vi "publish -- pll result.vi"(7 "publisher action":T4, 11 "pll result IN":T1={"freq (Hz)"=40017.438097734725, "gamma (Hz)"=0.0, "Voltage (V)"=6.817921124952451+0.0i, "overlimit ?"=FALSE, "running lorentzian out"={"A (VHz)"=-1.0311345636926572, "f (Hz)"=-1.0311345636926572, "G (Hz)"=-1.0311345636926572, "phi(rad)"=-1.0311345636926572, "Q"=-1.0311345636926572, "Norm  Ampl"=-1.0311345636926572, "bg (V)"=-1.0311345636926572+0.0i, "4corners"={"z (-pi/2)"=-1.0311345636926572+0.5736824521422934i, "z(inf)"=-0.5200164984937075+1.0975277942502903i, "z (pi/2)"=-1.0311345636926572+0.5736824521422934i, "z center"=-0.5136528600391839+0.580046090596817i, "z(0)"=-0.5200164984937075+1.0975277942502903i, "radius"=-1.0311345636926572}}, "static lorentzian out"={"A (VHz)"=6.817921124952451, "f (Hz)"=-1.0311345636926572, "G (Hz)"=-1.0311345636926572, "phi(rad)"=-1.0311345636926572, "Q"=-1.0311345636926572, "Norm  Ampl"=-1.0311345636926572, "bg (V)"=-1.0311345636926572+0.0i, "4corners"={"z (-pi/2)"=-1.0311345636926572+0.5736824521422934i, "z(inf)"=-0.5200164984937075+1.0975277942502903i, "z (pi/2)"=-1.0311345636926572+0.5736824521422934i, "z center"=-0.5136528600391839+0.580046090596817i, "z(0)"=-0.5200164984937075+1.0975277942502903i, "radius"=-1.0311345636926572}}} {"static lorentzian out"."bg (V)" format="%#9_9f"; "static lorentzian out"."Q" format="%#9_9f"; "static lorentzian out"."phi(rad)" format="%#9_9f"; "static lorentzian out"."G (Hz)" format="%#9_9f"; "static lorentzian out"."f (Hz)" format="%#9_9f"; "running lorentzian out"."bg (V)" format="%#9_9f"; "running lorentzian out"."Q" format="%#9_9f"; "running lorentzian out"."phi(rad)" format="%#9_9f"; "running lorentzian out"."G (Hz)" format="%#9_9f"; "running lorentzian out"."f (Hz)" format="%#9_9f"; "Voltage (V)" format="%#.4f"; "gamma (Hz)" format="%#.4f"; "freq (Hz)" format="%#.11f"}) -> (3 "pll result OUT":T1={"freq (Hz)"=40017.438097734725, "gamma (Hz)"=0.0, "Voltage (V)"=6.817921124952451+0.0i, "overlimit ?"=FALSE, "running lorentzian out"={"A (VHz)"=-1.0311345636926572, "f (Hz)"=-1.0311345636926572, "G (Hz)"=-1.0311345636926572, "phi(rad)"=-1.0311345636926572, "Q"=-1.0311345636926572, "Norm  Ampl"=-1.0311345636926572, "bg (V)"=-1.0311345636926572+0.0i, "4corners"={"z (-pi/2)"=-1.0311345636926572+0.5736824521422934i, "z(inf)"=-0.5200164984937075+1.0975277942502903i, "z (pi/2)"=-1.0311345636926572+0.5736824521422934i, "z center"=-0.5136528600391839+0.580046090596817i, "z(0)"=-0.5200164984937075+1.0975277942502903i, "radius"=-1.0311345636926572}}, "static lorentzian out"={"A (VHz)"=6.817921124952451, "f (Hz)"=-1.0311345636926572, "G (Hz)"=-1.0311345636926572, "phi(rad)"=-1.0311345636926572, "Q"=-1.0311345636926572, "Norm  Ampl"=-1.0311345636926572, "bg (V)"=-1.0311345636926572+0.0i, "4corners"={"z (-pi/2)"=-1.0311345636926572+0.5736824521422934i, "z(inf)"=-0.5200164984937075+1.0975277942502903i, "z (pi/2)"=-1.0311345636926572+0.5736824521422934i, "z center"=-0.5136528600391839+0.580046090596817i, "z(0)"=-0.5200164984937075+1.0975277942502903i, "radius"=-1.0311345636926572}}} {"static lorentzian out"."bg (V)" format="%#9_9f"; "static lorentzian out"."Q" format="%#9_9f"; "static lorentzian out"."phi(rad)" format="%#9_9f"; "static lorentzian out"."G (Hz)" format="%#9_9f"; "static lorentzian out"."f (Hz)" format="%#9_9f"; "running lorentzian out"."bg (V)" format="%#9_9f"; "running lorentzian out"."Q" format="%#9_9f"; "running lorentzian out"."phi(rad)" format="%#9_9f"; "running lorentzian out"."G (Hz)" format="%#9_9f"; "running lorentzian out"."f (Hz)" format="%#9_9f"; "Voltage (V)" format="%#.4f"; "gamma (Hz)" format="%#.4f"; "freq (Hz)" format="%#.11f"})   [LabVIEW 2020]
uses:
  pll talkback data type.ctl
  lorentzian.ctl
  circle corners.ctl
  publisher action.ctl
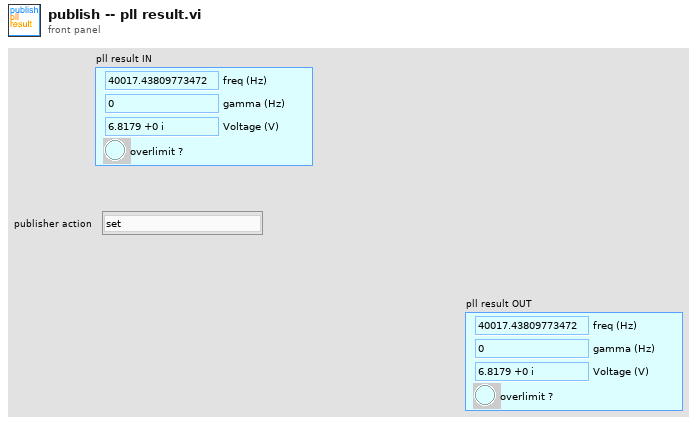
[diagram p1: front panel]
types:
  T1 = typedef "pll talkback data type.ctl" = cluster{"freq (Hz)":dbl, "gamma (Hz)":dbl, "Voltage (V)":cdb, "overlimit ?":bool, "running lorentzian out":T2, "static lorentzian out":T2}
  T2 = typedef "lorentzian.ctl" = cluster{"A (VHz)":dbl, "f (Hz)":dbl, "G (Hz)":dbl, "phi(rad)":dbl, "Q":dbl, "Norm  Ampl":dbl, "bg (V)":cdb, "4corners":T3}
  T3 = typedef "circle corners.ctl" = cluster{"z (-pi/2)":cdb, "z(inf)":cdb, "z (pi/2)":cdb, "z center":cdb, "z(0)":cdb, "radius":dbl}
  T4 = typedef "publisher action.ctl" = enum16{"set", "get", "init", "check"}
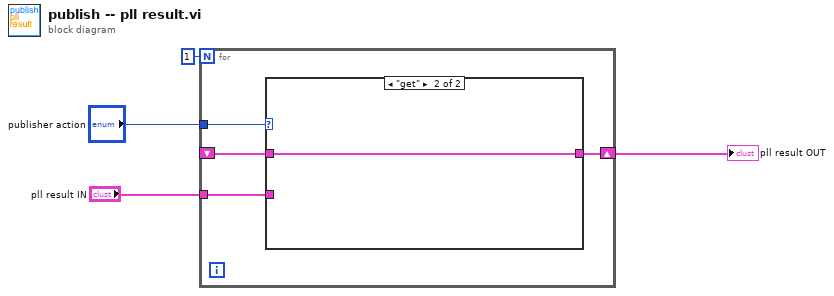
[diagram p0: block diagram]
diagram:
  n1 = for {
    N: 1 -> [_]
    tunnel: "publisher action" -> [w8]
    tunnel: "pll result IN" -> [w6]
    shift-right: [w7] -> w1
    shift-left: _ -> [w5]
    n2 = case shown="\"get\"" w8 {
      tunnel: [w9 w10] -> w7
      tunnel: w6 -> [w9 _]
      tunnel: w5 -> [_ w10]
      frame "set", Default {
      }
      frame "get" {
      }
    }
  }
  "pll result OUT" <- w1
